vi "Configure Display Layout.vi"(7 "Channel (1)":i32=1, 8 "error in (no error)":errorcluster, 10 "Graph Layout (0:D1)":u16(ring) items=["D1", "D12", "D1_2", "D112", "D1_1_2", "D123", "D1_2_3", "D12_33", "D11_23", "D13_23", "D12_13", "D1234", "D1_2_3_4", "D12_34", "D123_456", "D12_34_56", "D1234_5678", "D12_34_56_78", "D123_456_789", "D123_ABC", "D1234_9ABC", "D123_CDEF"], 11 "VISA resource name":refnum<visa-resource-name>) -> (0 "error out":errorcluster, 3 "VISA resource name out":refnum<visa-resource-name>)   [LabVIEW 2022 SP3, in "Agilent ENA Series.lvlib"]
doc: "Configures the graph layout for selected channel or the layout of the windows on the LCD display.\n\nNote:\nFor E5080A and E5080B models, if D1 is selected it is converted to channel/window layout. For the other parameters, it is converted to trace/window layout."
uses:
  <instrlib>/Agilent ENA Series/Agilent ENA Series.lvlib
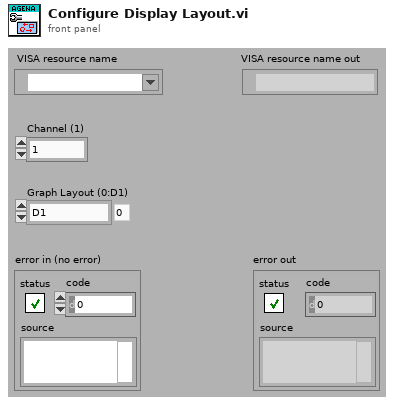
[diagram p1: front panel]
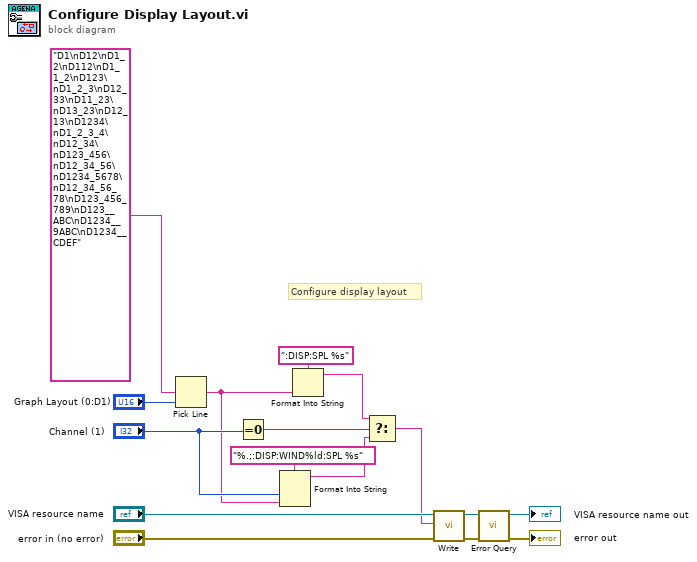
[diagram p0: block diagram]
diagram:
  # "Configure display layout"
  n1 = Pick Line(multi-line string="D1\nD12\nD1_2\nD112\nD1_1_2\nD123\nD1_2_3\nD12_33\nD11_23\nD13_23\nD12_13\nD1234\nD1_2_3_4\nD12_34\nD123_456\nD12_34_56\nD1234_5678\nD12_34_56_78\nD123_456_789\nD123__ABC\nD1234__9ABC\nD1234__CDEF", line index="Graph Layout (0:D1)") -> (output string=w8:string)  [unwired: 1 in]
  n2 = Equal To 0?(x="Channel (1)") -> (x = 0?=w13:bool)
  n3 = Format Into String(format string="%.;:DISP:WIND%ld:SPL %s", "Channel (1)", w8) -> (resulting string=w6:string)  [unwired: 2 in, 1 out]
  n4 = Format Into String(format string=":DISP:SPL %s", w8) -> (resulting string=w7:string)  [unwired: 2 in, 1 out]
  n5 = Select(t=w7, s=w13, f=w6) -> (s? t:f=w5:string)
  n6 = call <instrlib>:"Write.vi"("error in (no error)"="error in (no error)", "String ()"=w5, "VISA resource name"="VISA resource name") -> ("error out"=w3:errorcluster, "VISA resource name out"=w4:refnum<visa-resource-name>)  [unwired: 6 in, 1 out]
  n7 = call <instrlib>:"Error Query.vi"("error in (no error)"=w3, "VISA resource name"=w4) -> ("error out"=→"error out":errorcluster, "VISA resource name out"=→"VISA resource name out":refnum<visa-resource-name>)  [unwired: 6 in, 2 out]
